vi "Execute User Query.vi"(4 "error in (no error)":errorcluster, 5 "Return Data? (f)":bool, 6 "User Query":string, 7 "Statement Refnum":T1) -> (0 "error out":errorcluster, 1 "Data Present?":bool, 2 "Number of Columns":i32, 3 "Statement Refnum":T1)   [LabVIEW 2011]
doc: "Appelle la requête ACCESS et l'éxécute en tenant compte des paramètres chargés"
uses:
  SQL Controls/Statement Refnum.ctl
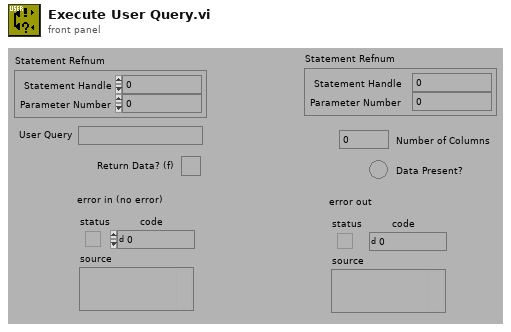
[diagram p1: front panel]
types:
  T1 = typedef "Statement Refnum.ctl" = cluster{"Statement Handle":i32, "Parameter Number":u16}
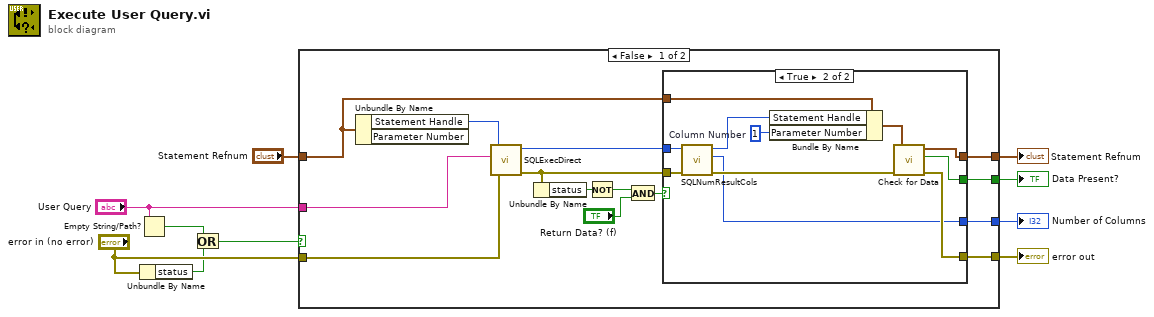
[diagram p0: block diagram]
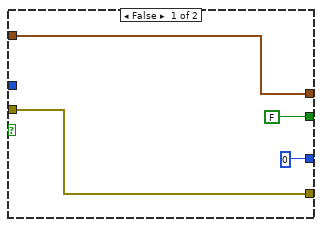
[diagram p2: hidden frame]
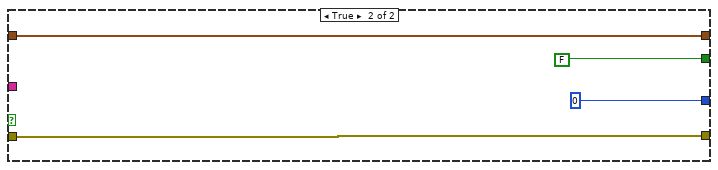
[diagram p3: hidden frame]
diagram:
  n1 = Empty String/Path?(string/path="User Query") -> (empty?=w3:bool)
  n2 = Unbundle By Name("error in (no error)") -> ("status"=w1:bool)
  n3 = Or(x=w3, y=w1) -> (x .or. y?=w2:bool)
  n4 = case shown="False" w2 {
    tunnel: "Statement Refnum" -> [w14 w43]
    tunnel: [w24 w43] -> w9
    tunnel: [w23 FALSE] -> w8
    tunnel: "error in (no error)" -> [w12 w42]
    tunnel: [w22 w42] -> w6
    tunnel: [w18 0] -> w5
    tunnel: "User Query" -> [w11 _]
    frame False {
      n5 = Unbundle By Name(w14) -> ("Statement Handle"=w13:i32)  [unwired: 1 out]
      n6 = call "SQLExecDirect.vi"("error in (no error)"=w12, "StatementText"=w11, "InputHandle"=w13) -> ("error out"=w15:errorcluster, "OutputHandle"=w16:i32)  [unwired: 3 out]
      n7 = Unbundle By Name(w15) -> ("status"=w19:bool)
      n8 = Not(x=w19) -> (.not. x?=w17:bool)
      n9 = And(x=w17, y="Return Data? (f)") -> (x .and. y?=w21:bool)
      n10 = case shown="True" w21 {
        tunnel: [w25 w39] -> w24
        tunnel: [FALSE w38] -> w23
        tunnel: [w26 w37] -> w22
        tunnel: w16 -> [_ w36]
        tunnel: w15 -> [w26 w35]
        tunnel: [0 w33] -> w18
        tunnel: w14 -> [w25 w32]
        frame False {
        }
        frame True {
          w30 = u16 1  # Column Number
          n11 = call "SQLNumResultCols.vi"("error in (no error)"=w35, "InputHandle"=w36) -> ("error out"=w34:errorcluster, "NumResultCols"=w33:i32, "OutputHandle"=w29:i32)  [unwired: 3 out]
          n12 = Bundle By Name(cluster=w32, "Statement Handle"=w29, "Parameter Number"=w30) -> (w31:T1)
          n13 = call "Check for Data.vi"("error in (no error)"=w34, "Statement Refnum"=w31) -> ("error out"=w37:errorcluster, "Data Present?"=w38:bool, "Statement Refnum"=w39:T1)  [unwired: 3 out]
        }
      }
    }
    frame True {
    }
  }
  "Statement Refnum" <- w9
  "Data Present?" <- w8
  "error out" <- w6
  "Number of Columns" <- w5
